vi "BotSpeakTCP_WriteRead1.vi"(4 "error in":errorcluster, 5 "To Send":string, 6 "connection ID":refnum<k5>, 7 "Timeout":i32) -> (0 "error out":errorcluster, 1 "data out":string, 2 "connection ID out":refnum<k5>)   [LabVIEW 2012]
uses:
  <userlib>/botspeak/VIs/SubVIs/BotSpeak_Globals.vi
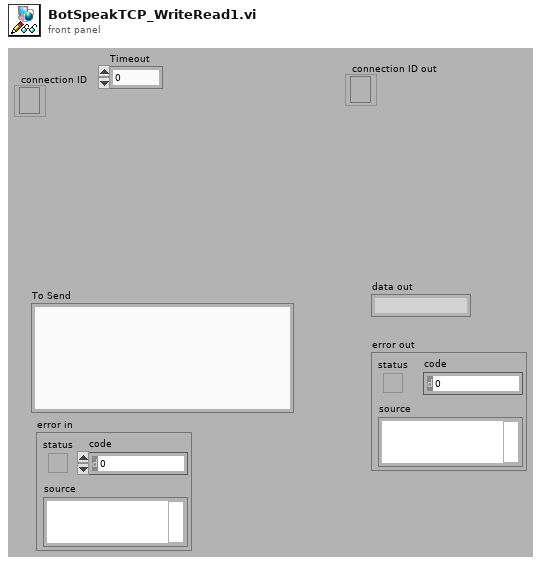
[diagram p1: front panel]
types:
  T1 = enum16{"Standard", "Buffered", "CRLF", "Immediate"}
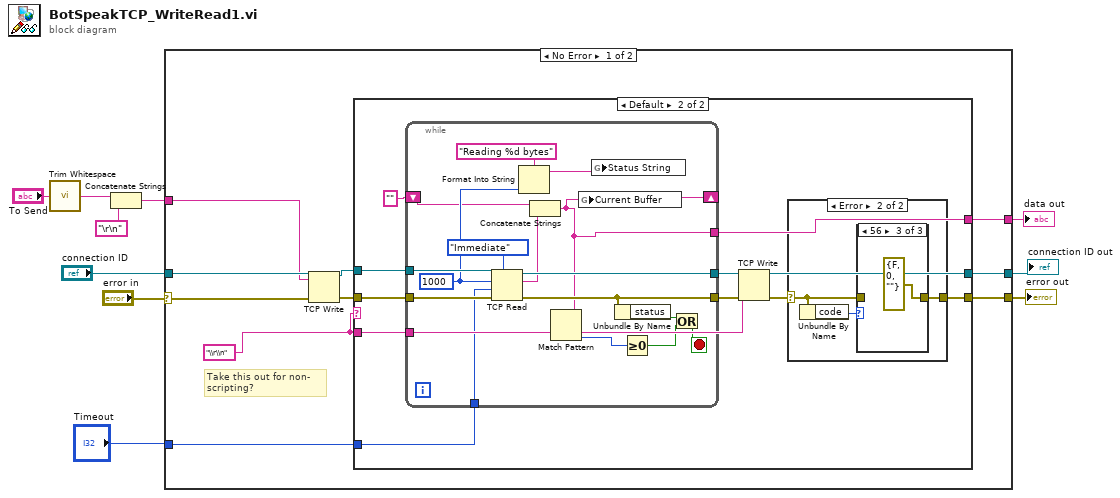
[diagram p0: block diagram]
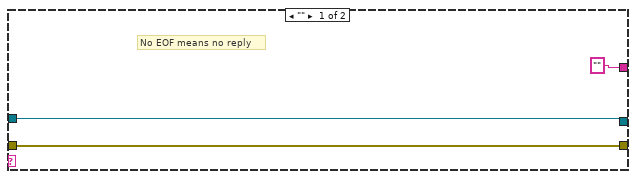
[diagram p2: hidden frame]
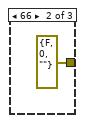
[diagram p5: hidden frame]
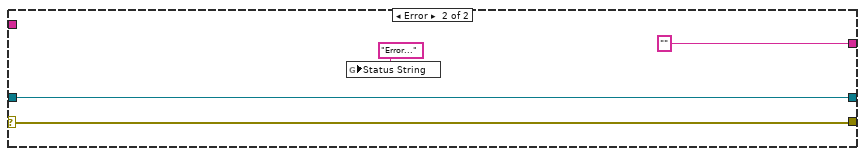
[diagram p6: hidden frame]
diagram:
  n1 = call <vilib>:"Trim Whitespace.vi"("string"="To Send") -> ("trimmed string"=w2:string)  [unwired: 1 in]
  n2 = Concatenate Strings(w2, "\r\n" ("string")) -> (w5:string)
  n3 = case shown="No Error" "error in" {
    selector: "error in" -> [w17 w60]
    tunnel: [w20 ""] -> w7
    tunnel: [w19 w60] -> w8
    tunnel: "connection ID" -> [w18 w59]
    tunnel: w5 -> [w14 _]
    tunnel: [w13 w59] -> w4
    tunnel: "Timeout" -> [w12 _]
    frame No Error {
      w11 = "\\r\\n" ("Reply EOF")
      # "Take this out for non-\nscripting?"
      n4 = TCP Write(connection ID=w18, data in=w14, error in (no error)=w17) -> (connection ID out=w15:refnum<k5>, error out=w16:errorcluster)  [unwired: 1 in, 1 out]
      n5 = case shown="Default" w11 {
        tunnel: w11 -> [_ w27]
        tunnel: ["" w26] -> w20
        tunnel: [w22 w24] -> w19
        tunnel: w15 -> [w21 w34]
        tunnel: w16 -> [w22 w33]
        tunnel: w12 -> [_ w30]
        tunnel: [w21 w29] -> w13
        frame "" {
          # "No EOF means no reply"
        }
        frame Default {
          n6 = while {
            tunnel: w34 -> [w58]
            tunnel: w33 -> [w57]
            tunnel: [w54] -> w32
            tunnel: [w45] -> w31
            tunnel: w30 -> [w51]
            shift-right: [w42] -> _
            shift-left: "" ("data out") -> [w50]
            tunnel: w27 -> [w48]
            tunnel: [w42] -> w26
            stop <- w43 stop-if-true
            w52 = 1000 ("bytes to read")
            n7 = TCP Read(connection ID=w58, bytes to read=w52, error in (no error)=w57, 7:T1."Immediate" ("mode (standard)"), 9:w51) -> (connection ID out=w54:refnum<k5>, data out=w49:string, error out=w45:errorcluster)
            n8 = Format Into String(format string="Reading %d bytes", w52) -> (resulting string=w55:string)  [unwired: 2 in, 1 out]
            n9 = Concatenate Strings(w50, w49) -> (w42:string)
            n10 = Match Pattern(string=w42, regular expression=w48) -> (offset past match=w47:i32)  [unwired: 1 in, 3 out]
            n11 = global write "BotSpeak_Globals.vi" "Current Buffer"(w42) -> ()
            n12 = global write "BotSpeak_Globals.vi" "Status String"(w55) -> ()
            n13 = Unbundle By Name(w45) -> ("status"=w44:bool)
            n14 = Greater Or Equal To 0?(x=w47) -> (x >= 0?=w46:bool)
            n15 = Or(x=w44, y=w46) -> (x .or. y?=w43:bool)
          }
          n16 = TCP Write(connection ID=w32, data in=w27, error in (no error)=w31) -> (connection ID out=w29:refnum<k5>, error out=w25:errorcluster)  [unwired: 1 in, 1 out]
          n17 = case shown="Error" w25 {
            selector: w25 -> [w35 w36]
            tunnel: [w35 w37] -> w24
            frame No Error {
            }
            frame Error {
              n18 = Unbundle By Name(w36) -> ("code"=w38:i32)
              n19 = case shown="56" w38 {
                tunnel: [w39 errorcluster {"status"=FALSE, "code"=0, "source"=""} ("error IO") errorcluster {"status"=FALSE, "code"=0, "source"=""} ("error IO")] -> w37
                tunnel: w36 -> [w39 _ _]
                frame Default {
                }
                frame 66 {
                }
                frame 56 {
                }
              }
            }
          }
        }
      }
    }
    frame Error {
      n20 = global write "BotSpeak_Globals.vi" "Status String"("Error..." ("Status String")) -> ()
    }
  }
  "error out" <- w8
  "data out" <- w7
  "connection ID out" <- w4
